vi "CreateTypedef.vi"(8 "error in (no error)":errorcluster, 11 "Message in":T1) -> (0 "error out":errorcluster, 3 "Message out":T1)   [LabVIEW 2017, in "MessageGen.lvlib"]
uses:
  <vilib>/addons/InsightCM/MessageBus/CodeGen/MessageGen.lvlib
  <vilib>/addons/InsightCM/MessageBus/CodeGen/controls/MessageData.ctl
  <vilib>/addons/InsightCM/MessageBus/CodeGen/controls/MessageType.ctl
  <vilib>/addons/InsightCM/MessageBus/CodeGen/controls/Parameter.ctl
  <vilib>/addons/InsightCM/MessageBus/CodeGen/controls/ParameterType.ctl
  <vilib>/LabVIEW Icon API/API_Text.ctl
  <vilib>/LabVIEW Icon API/LabVIEW Icon API.lvlib
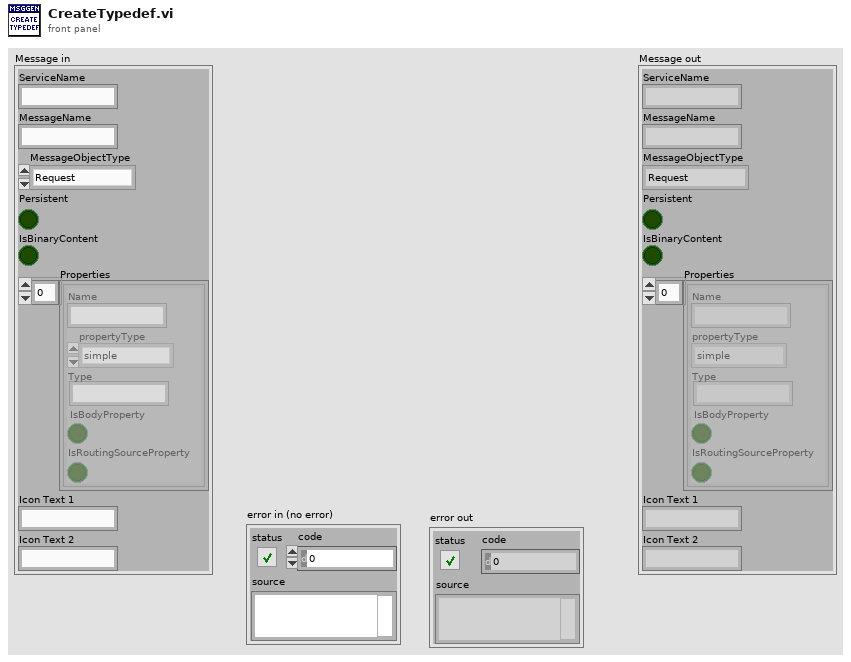
[diagram p1: front panel]
types:
  T1 = typedef "MessageGen.lvlib/MessageData.ctl" = cluster{"ServiceName":string, "MessageName":string, "MessageObjectType":T2, "Persistent":bool, "IsBinaryContent":bool, "Properties":T3[], "Icon Text 1":string, "Icon Text 2":string}
  T2 = typedef "MessageGen.lvlib/MessageType.ctl" = enum16{"Request", "Response", "Broadcast", "RoutedMessage"}
  T3 = typedef "MessageGen.lvlib/Parameter.ctl" = cluster{"Name":string, "propertyType":T4, "Type":string, "IsBodyProperty":bool, "IsRoutingSourceProperty":bool}
  T4 = typedef "MessageGen.lvlib/ParameterType.ctl" = enum16{"simple", "bytearray", "dateTime", "list", "map", "object"}
  T5 = typedef "LabVIEW Icon API.lvlib/API_Text.ctl" = cluster{"Line 1 text":string, "Line 2 text":string, "Line 3 text":string, "Line 4 text":string}
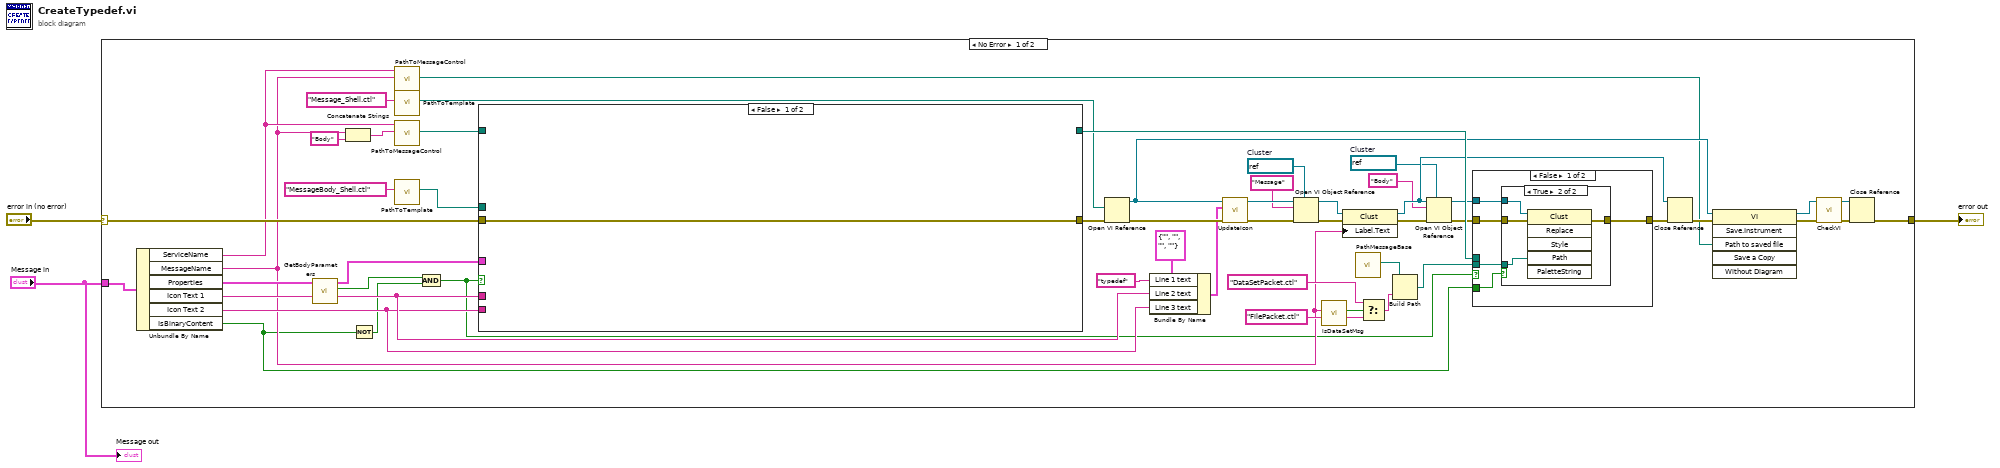
[diagram p0: block diagram]
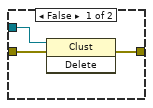
[diagram p2: hidden frame]
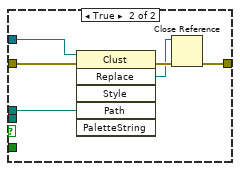
[diagram p3: hidden frame]
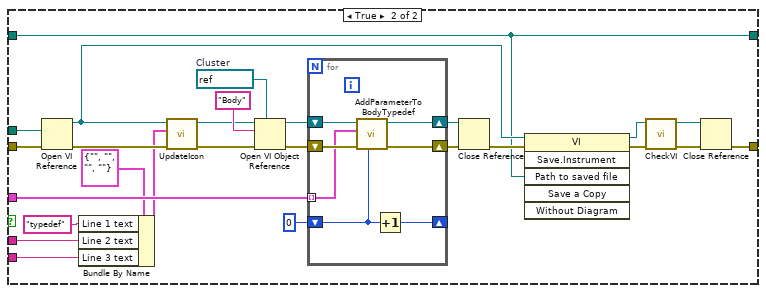
[diagram p4: hidden frame]
diagram:
  n1 = case shown="No Error" "error in (no error)" {
    selector: "error in (no error)" -> [w54 w108]
    tunnel: [w55 w108] -> w2
    tunnel: "Message in" -> [w31 _]
    frame No Error {
      w41 = refnum<vi> refnum  # Cluster
      w49 = refnum<vi> refnum  # Cluster
      n2 = Unbundle By Name(w31) -> ("ServiceName"=w21:string, "MessageName"=w9:string, "Properties"=w27:T3[], "Icon Text 1"=w14:string, "Icon Text 2"=w13:string, "IsBinaryContent"=w7:bool)
      n3 = call <vilib>:"GetBodyParameters.vi"("Parameters"=w27) -> ("HasBodyParameters"=w5:bool, "BodyParameters"=w26:T3[])  [unwired: 9 in]
      n4 = Concatenate Strings(w9, "Body" ("string")) -> (w23:string)
      n5 = Not(x=w7) -> (.not. x?=w6:bool)
      n6 = call <vilib>:"PathToMessageControl.vi"("ControlName"=w9, "Service"=w21) -> ("Path"=w20:path)  [unwired: 9 in]
      n7 = call <vilib>:"PathToTemplate.vi"("TemplateName"="Message_Shell.ctl") -> ("Path"=w29:path)  [unwired: 10 in]
      n8 = call <vilib>:"PathToMessageControl.vi"("ControlName"=w23, "Service"=w21) -> ("Path"=w24:path)  [unwired: 9 in]
      n9 = call <vilib>:"PathToTemplate.vi"("TemplateName"="MessageBody_Shell.ctl") -> ("Path"=w28:path)  [unwired: 10 in]
      n10 = And(x=w5, y=w6) -> (x .and. y?=w4:bool)
      n11 = case shown="False" w4 {
        tunnel: w24 -> [_ w80]
        tunnel: w28 -> [_ w95]
        tunnel: w54 -> [w74 w94]
        tunnel: [w74 w93] -> w48
        tunnel: w14 -> [_ w75]
        tunnel: w26 -> [_ w83]
        tunnel: [_ w80] -> w45
        tunnel: w13 -> [_ w76]
        frame False {
        }
        frame True {
          w97 = refnum<vi> refnum  # Cluster
          n12 = Open VI Reference(vi path=w95, error in (no error)=w94) -> (vi reference=w86:refnum<vi>, error out=w88:errorcluster)  [unwired: 4 in]
          n13 = Bundle By Name(cluster=T5 {"Line 1 text"="", "Line 2 text"="", "Line 3 text"="", "Line 4 text"=""} ("Text"), "Line 1 text"="typedef" ("method"), "Line 2 text"=w75, "Line 3 text"=w76) -> (w78:T5)
          n14 = call <vilib>:"UpdateIcon.vi"("error in (no error)"=w88, "Text"=w78, "VI Refnum in"=w86) -> ("error out"=w87:errorcluster, "VI Refnum out"=w85:refnum<vi>)  [unwired: 7 in]
          n15 = Open VI Object Reference(7:w97, 8:w87, 10:"Body" ("name/order"), 11:w85) -> (0:w81:errorcluster, 3:w82:refnum<vi>)
          n16 = for {
            tunnel: w83 -> [w102] mode=indexing
            shift-right: [w106] -> _
            shift-left: 0 -> [w107]
            shift-right: [w103] -> w100
            shift-left: w81 -> [w104]
            shift-right: [w101] -> w84
            shift-left: w82 -> [w105]
            n17 = call <vilib>:"AddParameterToBodyTypedef.vi"("Number of Parameters already added"=w107, "error in (no error)"=w104, "Property"=w102, "Clust Refnum"=w105) -> ("error out"=w103:errorcluster, "Cluster Ref out"=w101:refnum<vi>)  [unwired: 6 in]
            n18 = Increment(x=w107) -> (x+1=w106:i32)
          }
          n19 = Close Reference(reference=w84, error in (no error)=w100) -> (error out=w98:errorcluster)
          n20 = invoke class="VI" method="Save.Instrument"(reference=w86, error in=w98, "Path to saved file"=w80) -> (reference out=w89:refnum<vi>, error out=w90:errorcluster)  [unwired: 3 in, 4 out]
          n21 = call <vilib>:"CheckVI.vi"("error in (no error)"=w90, "VI ref"=w89) -> ("error out"=w92:errorcluster, "VI ref out"=w91:refnum<vi>)  [unwired: 8 in]
          n22 = Close Reference(reference=w91, error in (no error)=w92) -> (error out=w93:errorcluster)
        }
      }
      n23 = Open VI Reference(vi path=w29, error in (no error)=w48) -> (vi reference=w42:refnum<vi>, error out=w51:errorcluster)  [unwired: 4 in]
      n24 = Bundle By Name(cluster=T5 {"Line 1 text"="", "Line 2 text"="", "Line 3 text"="", "Line 4 text"=""} ("Text"), "Line 1 text"="typedef" ("method"), "Line 2 text"=w14, "Line 3 text"=w13) -> (w15:T5)
      n25 = call <vilib>:"UpdateIcon.vi"("error in (no error)"=w51, "Text"=w15, "VI Refnum in"=w42) -> ("error out"=w52:errorcluster, "VI Refnum out"=w53:refnum<vi>)  [unwired: 7 in]
      n26 = Open VI Object Reference(7:w49, 8:w52, 10:"Message" ("name/order"), 11:w53) -> (0:w46:errorcluster, 3:w47:refnum<vi>)
      n27 = call <vilib>:"IsDataSetMsg.vi"("MessageName"=w9) -> ("IsDataSet"=w8:bool)  [unwired: 10 in]
      n28 = property class="Clust"(reference=w47, error in=w46, "Label.Text"=w9) -> (reference out=w43:refnum<vi>, error out=w44:errorcluster)
      n29 = call <vilib>:"PathMessageBase.vi"() -> ("Path"=w19:path)  [unwired: 11 in]
      n30 = Select(t="DataSetPacket.ctl" ("name or relative path"), s=w8, f="FilePacket.ctl" ("name or relative path")) -> (s? t:f=w10:string)
      n31 = Build Path(base path=w19, name or relative path=w10) -> (appended path=w18:path)
      n32 = Open VI Object Reference(7:w41, 8:w44, 10:"Body" ("name/order"), 11:w43) -> (0:w38:errorcluster, 3:w39:refnum<vi>)
      n33 = case shown="False" w4 {
        tunnel: w45 -> [_ w73]
        tunnel: w39 -> [w60 w72]
        tunnel: w38 -> [w59 w71]
        tunnel: [w58 w69] -> w33
        tunnel: w7 -> [w57 _]
        tunnel: w18 -> [w56 _]
        frame False {
          n34 = case shown="True" w57 {
            tunnel: w60 -> [w63 w65]
            tunnel: w59 -> [w62 w67]
            tunnel: [w61 w66] -> w58
            tunnel: w56 -> [_ w64]
            frame False {
              n35 = invoke class="Clust" method="Delete"(reference=w63, error in=w62) -> (error out=w61:errorcluster)  [unwired: 1 in, 2 out]
            }
            frame True {
              n36 = invoke class="Clust" method="Replace"(reference=w65, error in=w67, "Path"=w64) -> (error out=w66:errorcluster)  [unwired: 3 in, 5 out]
            }
          }
        }
        frame True {
          n37 = invoke class="Clust" method="Replace"(reference=w72, error in=w71, "Path"=w73) -> (error out=w70:errorcluster, "Replace"=w68:refnum<vi>)  [unwired: 3 in, 4 out]
          n38 = Close Reference(reference=w68, error in (no error)=w70) -> (error out=w69:errorcluster)
        }
      }
      n39 = Close Reference(reference=w43, error in (no error)=w33) -> (error out=w32:errorcluster)
      n40 = invoke class="VI" method="Save.Instrument"(reference=w42, error in=w32, "Path to saved file"=w20) -> (reference out=w37:refnum<vi>, error out=w36:errorcluster)  [unwired: 3 in, 4 out]
      n41 = call <vilib>:"CheckVI.vi"("error in (no error)"=w36, "VI ref"=w37) -> ("error out"=w34:errorcluster, "VI ref out"=w35:refnum<vi>)  [unwired: 8 in]
      n42 = Close Reference(reference=w35, error in (no error)=w34) -> (error out=w55:errorcluster)
    }
    frame Error {
    }
  }
  "error out" <- w2
  "Message out" <- "Message in"
